vi "Write To DMA FIFO.vi"(8 "Error In":errorcluster, 10 "Data":u8[](array[numeric]), 11 "Display In":refnum<class "Neopixel - Host.lvclass">) -> (0 "Error Out":errorcluster, 3 "Display Out":refnum<class "Neopixel - Host.lvclass">)   [LabVIEW 2021, in "Neopixel - Host.lvclass"]
uses:
  Neopixel - Host.lvclass
  <vilib>/Utility/error.llb/Error Cluster From Error Code.vi
  <vilib>/rvi/errors/niLvFpgaAdjustHostInterfaceError.vi
  Public/Controls/FPGA Reference.ctl
  <vilib>/rvi/interface/nirviMethod/nirviMethod.xnode
  Neopixel - Host.lvclass/Neopixel - Host.ctl
  <vilib>/FPGAPlugInAG/Dynamic/niLvFpga_WriteFifo_Dynamic.vi
  <vilib>/rvi/errors/niLvFpgaMergeErrorWithErrorCode.vi
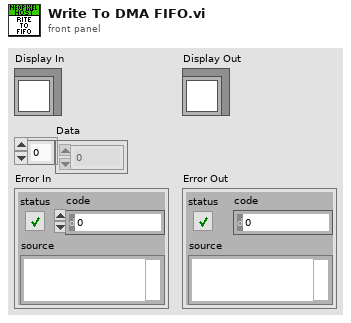
[diagram p1: front panel]
types:
  T1 = typedef "Neopixel - Host.lvclass/FPGA Reference.ctl" = refnum<k20>
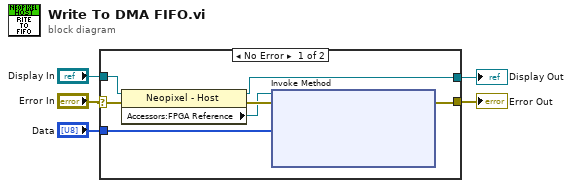
[diagram p0: block diagram]
diagram:
  n1 = case shown="No Error" "Error In" {
    selector: "Error In" -> [w11 w13]
    tunnel: [w12 w13] -> w5
    tunnel: "Display In" -> [w10 w14]
    tunnel: [w8 w14] -> w2
    tunnel: "Data" -> [w7 _]
    frame No Error {
      n2 = property class="Neopixel - Host"(reference=w10, error in=w11) -> (reference out=w8:refnum<class "Neopixel - Host.lvclass">, error out=w9:errorcluster, "Accessors:FPGA Reference"=w6:T1)
      n3 = xnode "Invoke Method"("FPGA VI Reference In"=w6, "error in"=w9, "Data"=w7) -> ("error out"=w12:errorcluster)  [unwired: 1 in, 2 out]
    }
    frame Error {
    }
  }
  "Display Out" <- w2
  "Error Out" <- w5
